vi "查找程序边框.vi"(11 "数组":string[][](array[string])) -> (0 "类型":string[](array[string]), 3 "边界":cluster{"左":i32, "上":i32, "右":i32, "下":i32}[](array[cluster]))   [LabVIEW 2020]
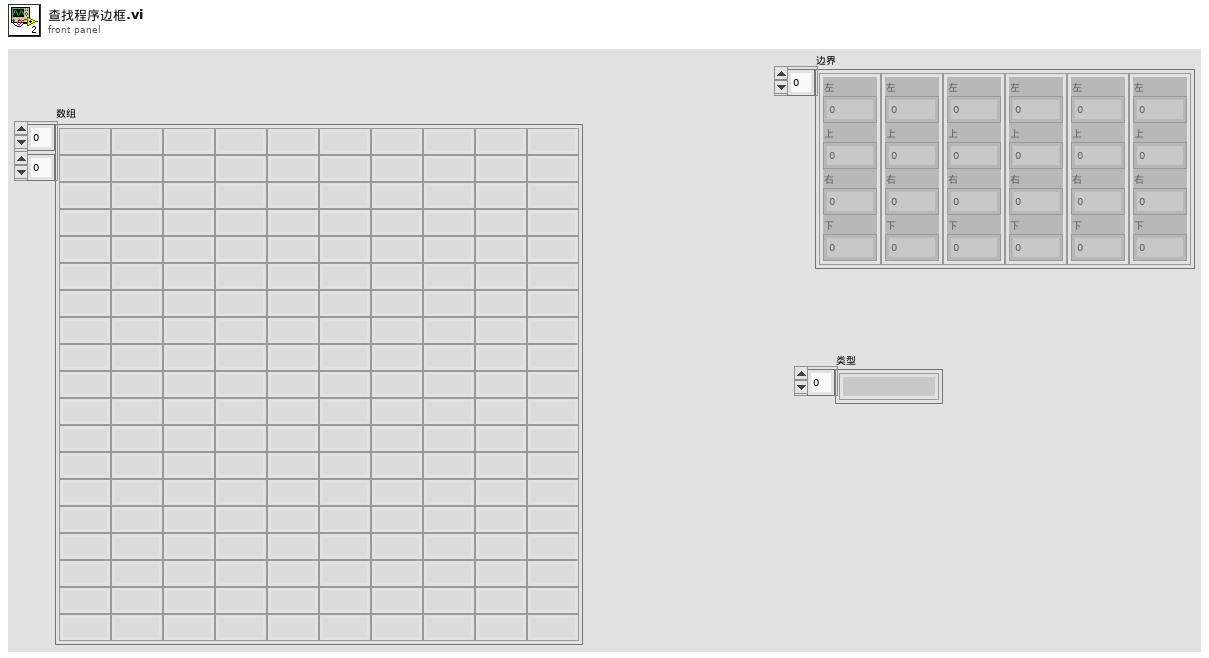
[diagram p1: front panel]
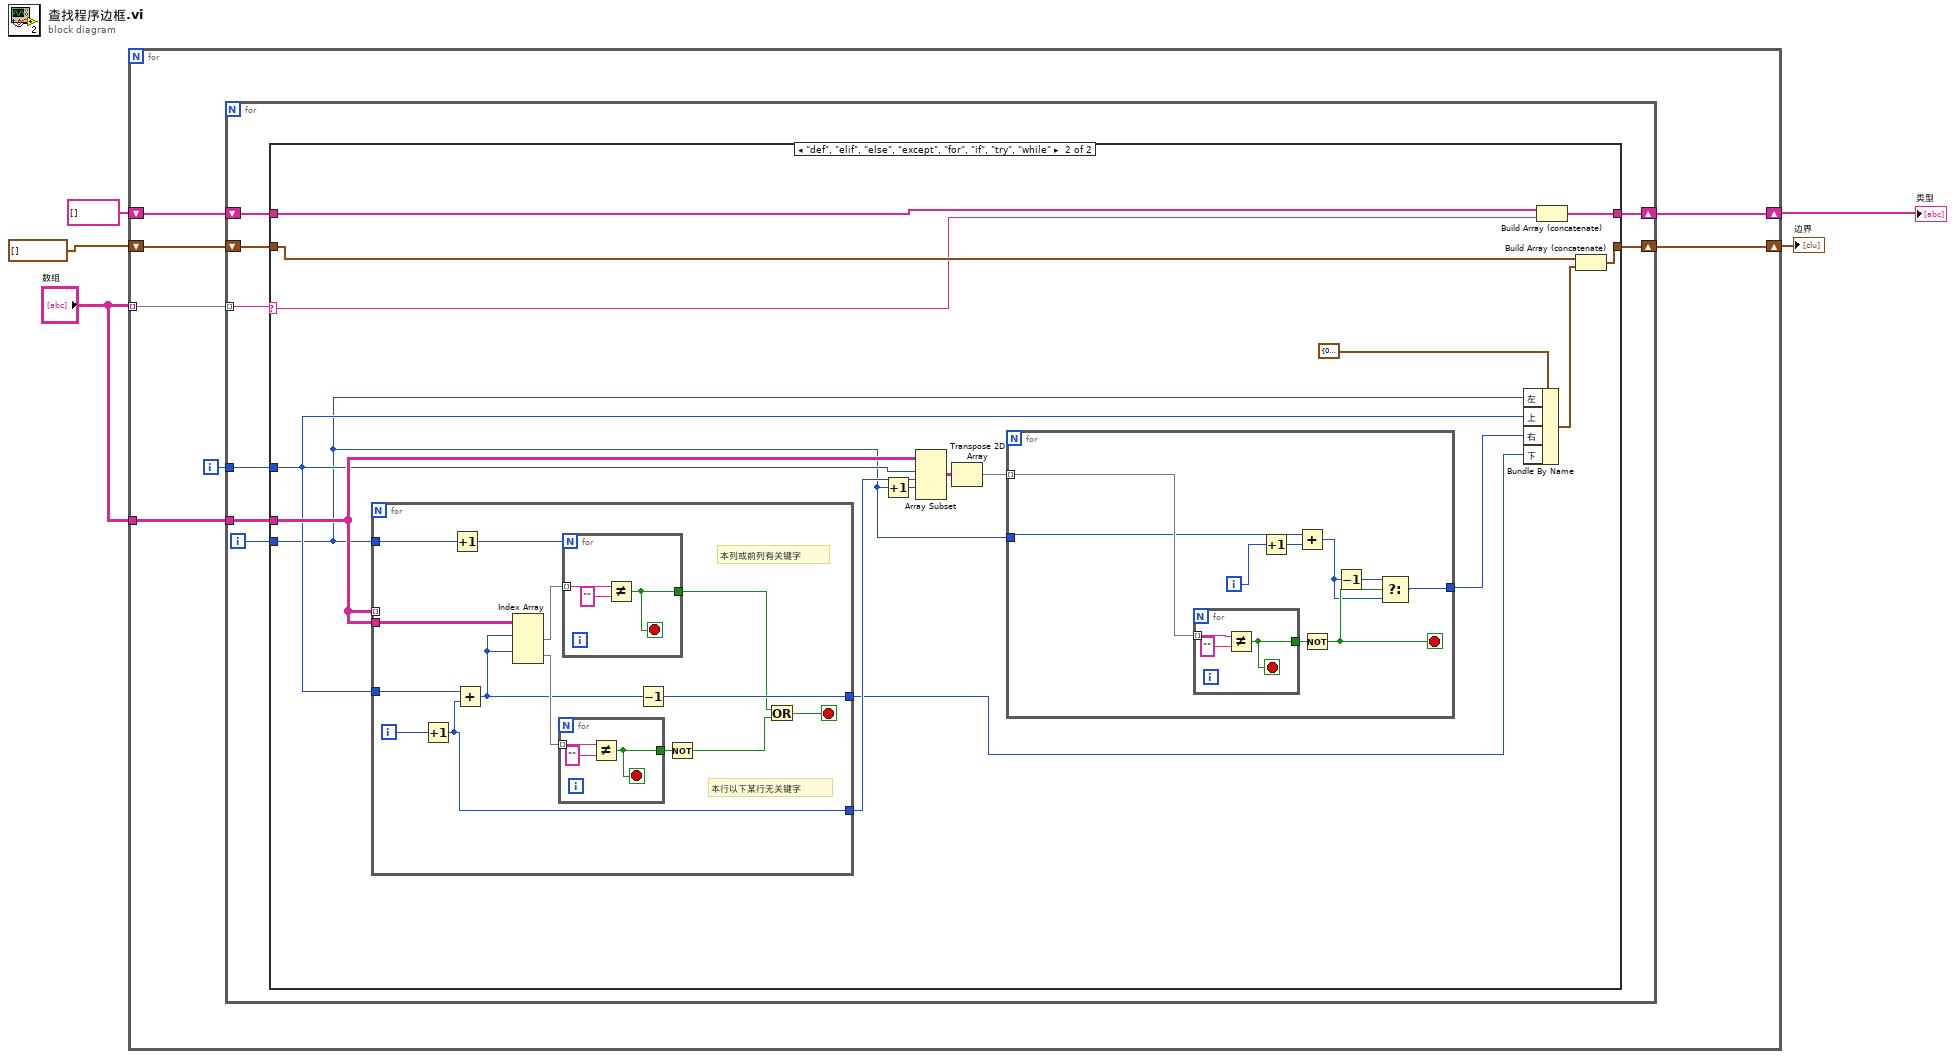
[diagram p0: block diagram]
diagram:
  n1 = for {
    tunnel: "数组" -> [w12] mode=indexing
    tunnel: "数组" -> [w10]
    shift-right: [w8] -> w3
    shift-left: cluster{"左":i32, "上":i32, "右":i32, "下":i32}[] [] -> [w9]
    shift-right: [w7] -> w1
    shift-left: string[] [] -> [w6]
    i -> [w11]
    n2 = for {
      tunnel: w12 -> [w20] mode=indexing
      tunnel: w11 -> [w18]
      tunnel: w10 -> [w17]
      shift-right: [w15] -> w8
      shift-left: w9 -> [w16]
      shift-right: [w14] -> w7
      shift-left: w6 -> [w13]
      i -> [w19]
      n3 = case shown="\"def\", \"elif\", \"else\", \"except\", \"for\", \"if\", \"try\", \"while\"" w20 {
        selector: w20 -> [_ w25]
        tunnel: w19 -> [_ w27]
        tunnel: w18 -> [_ w33]
        tunnel: w17 -> [_ w38]
        tunnel: w16 -> [w22 w30]
        tunnel: [w22 w28] -> w15
        tunnel: [w21 w24] -> w14
        tunnel: w13 -> [w21 w23]
        frame "假", Default {
        }
        frame "def", "elif", "else", "except", "for", "if", "try", "while" {
          n4 = for {
            tunnel: w38 -> [w64]
            tunnel: w33 -> [w62]
            tunnel: w38 -> [_] mode=indexing
            tunnel: w27 -> [w54]
            tunnel: [w55] -> w31
            tunnel: [w56] -> w37
            i -> [w63]
            stop <- w58 stop-if-true
            # "本行以下某行无关键字"
            # "本列或前列有关键字"
            n5 = Increment(x=w63) -> (x+1=w56:i32)
            n6 = Increment(x=w54) -> (x+1=w53:i32)
            n7 = Add(x=w62, y=w56) -> (x+y=w57:i32)
            n8 = Index Array(array=w64, index (row) #1=w57, index (row) #2=w57) -> (element #1=w52:string[], element #2=w61:string[])  [unwired: 2 in]
            n9 = for {
              tunnel: w61 -> [w70] mode=indexing
              tunnel: [w68] -> w60
              stop <- w68 stop-if-true
              n10 = Not Equal?(x=w70, y="") -> (x != y?=w68:bool)
            }
            n11 = for {
              N: w53 -> [_]
              tunnel: w52 -> [w67] mode=indexing
              tunnel: [w65] -> w51
              stop <- w65 stop-if-true
              n12 = Not Equal?(x=w67, y="") -> (x != y?=w65:bool)
            }
            n13 = Decrement(x=w57) -> (x-1=w55:i32)
            n14 = Not(x=w60) -> (.not. x?=w59:bool)
            n15 = Or(x=w51, y=w59) -> (x .or. y?=w58:bool)
          }
          n16 = Increment(x=w27) -> (x+1=w26:i32)
          n17 = Array Subset(array=w38, index (row)=w33, length (row)=w37, index (col)=w26) -> (w36:string[][])  [unwired: 1 in]
          n18 = Transpose 2D Array(2D array=w36) -> (transposed array=w35:string[][])
          n19 = for {
            tunnel: [w39] -> w32
            tunnel: w35 -> [w46] mode=indexing
            tunnel: w27 -> [w44]
            i -> [w45]
            stop <- w42 stop-if-true
            n20 = for {
              tunnel: [w49] -> w47
              tunnel: w46 -> [w48] mode=indexing
              stop <- w49 stop-if-true
              n21 = Not Equal?(x=w48, y="") -> (x != y?=w49:bool)
            }
            n22 = Increment(x=w45) -> (x+1=w43:i32)
            n23 = Add(x=w44, y=w43) -> (x+y=w41:i32)
            n24 = Not(x=w47) -> (.not. x?=w42:bool)
            n25 = Decrement(x=w41) -> (x-1=w40:i32)
            n26 = Select(t=w40, s=w42, f=w41) -> (s? t:f=w39:i32)
          }
          n27 = Bundle By Name(cluster=cluster{"左":i32, "上":i32, "右":i32, "下":i32} {"左"=0, "上"=0, "右"=0, "下"=0} ("输入簇"), "左"=w27, "上"=w33, "右"=w32, "下"=w31) -> (w29:cluster{"左":i32, "上":i32, "右":i32, "下":i32})
          n28 = Build Array (concatenate)(w23, w25) -> (w24:string[])
          n29 = Build Array (concatenate)(w30, w29) -> (w28:cluster{"左":i32, "上":i32, "右":i32, "下":i32}[])
        }
      }
    }
  }
  "边界" <- w3
  "类型" <- w1
